vi "session_callback_receive.vi"(8 "error in (no error)":errorcluster, 9 "flags":i32, 10 "length":u64, 11 "socket":u64) -> (0 "error out":errorcluster, 1 "buffer":u8[](array[numeric]), 2 "bytes received":i64)   [LabVIEW 2017]
doc: "Called when libssh2 wants to read data from the connection.\n\n<B>socket</B> the socket to read from.\n<B>length</B> number of bytes to read from the connection.\n<B>flags</B> flags that would have been used by a send() call.\n\nReturns the actual number of bytes received and the received bytes."
uses:
  ws2_32.dll
  libc.so.6
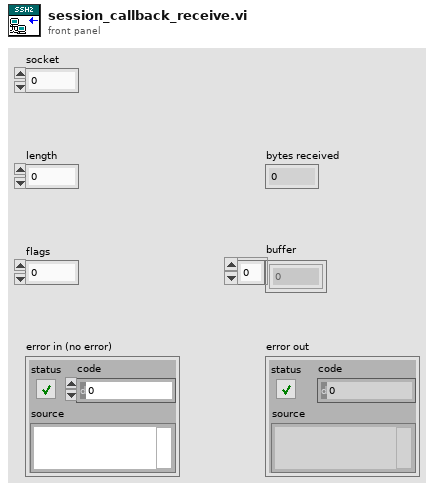
[diagram p1: front panel]
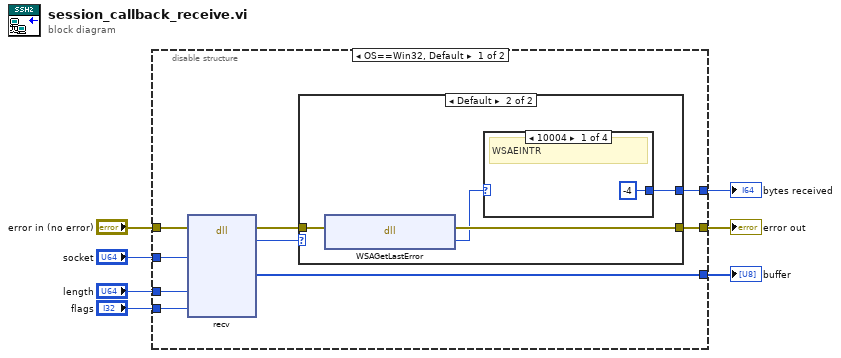
[diagram p0: block diagram]
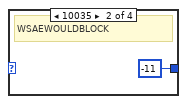
[diagram p3: hidden frame]
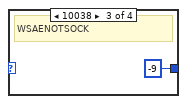
[diagram p4: hidden frame]
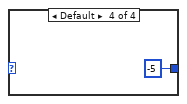
[diagram p5: hidden frame]
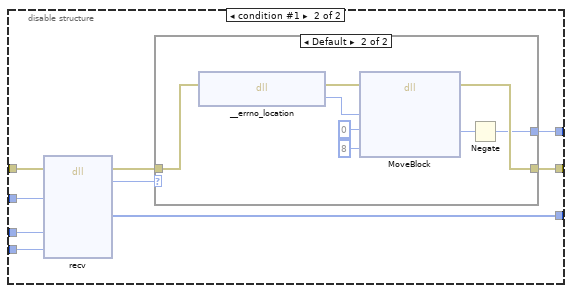
[diagram p6: hidden frame]
diagram:
  n1 = disable-structure shown="OS==Win32, Default" {
    disable-tunnel: "socket" -> [w16 w31]
    disable-tunnel: "length" -> [w15 w30]
    disable-tunnel: "flags" -> [w14 w29]
    disable-tunnel: "error in (no error)" -> [w13 w33]
    disable-tunnel: [w12 w28] -> w3
    disable-tunnel: [w10 w35] -> w2
    disable-tunnel: [w8 w34] -> w1
    frame condition #0 (active) {
      n2 = dll-call lib="ws2_32.dll" fn="recv"(error in=w13, "s"=w16, "len"=w15, "flags"=w14) -> (error out=w11:errorcluster, "return type"=w9:i32, "buf"=w12:u8[])  [unwired: 6 in, 1 out]
      n3 = case shown="Default" w9 {
        selector: w9 -> [w18 _]
        tunnel: w11 -> [w17 w22]
        tunnel: [w17 w21] -> w10
        tunnel: [w18 w19] -> w8
        frame 0.. {
        }
        frame Default {
          n4 = dll-call lib="ws2_32.dll" fn="WSAGetLastError"(error in=w22) -> (error out=w21:errorcluster, "return type"=w20:i32)  [unwired: 2 in, 1 out]
          n5 = case shown="10004" w20 {
            tunnel: [-4 -11 -9 -5] -> w19
            frame 10004 {
              # "WSAEINTR"
            }
            frame 10035 {
              # "WSAEWOULDBLOCK"
            }
            frame 10038 {
              # "WSAENOTSOCK"
            }
            frame Default {
            }
          }
        }
      }
    }
    frame condition #1 {
      n6 = dll-call lib="libc.so.6" fn="recv"(error in=w33, "sockfd"=w31, "size"=w30, "flags"=w29) -> (error out=w32:errorcluster, "return type"=w27:i32, "buf"=w28:u8[])  [unwired: 6 in, 1 out]
      n7 = case shown="Default" w27 {
        selector: w27 -> [w37 _]
        tunnel: w32 -> [w36 w45]
        tunnel: [w36 w42] -> w35
        tunnel: [w37 w38] -> w34
        frame 0.. {
        }
        frame Default {
          n8 = dll-call lib="libc.so.6" fn="__errno_location"(error in=w45) -> (error out=w43:errorcluster, "return type"=w41:u64)  [unwired: 2 in, 1 out]
          n9 = dll-call lib="LabVIEW" fn="MoveBlock"(error in=w43, "ps"=w41, "pd"=0, "size"=u64 8) -> (error out=w42:errorcluster, "pd"=w39:i32)  [unwired: 5 in, 1 out]
          n10 = Negate(x=w39) -> (-x=w38:i32)
        }
      }
    }
  }
  "error out" <- w2
  "buffer" <- w3
  "bytes received" <- w1
